vi "dfcg.vi"() -> ()   [LabVIEW 2020]
uses:
  <instrlib>/Lake Shore 372/Lake Shore 372.lvlib
panel:
  out "Quadrature Reading":dbl min=0.0 max=0.01 step=1e-05 format="%^.5e"
  out "Power Reading":dbl min=0.0 max=0.01 step=1e-05 format="%^.5e"
  out "Kelvin Reading":dbl min=0.0 max=1000.0 step=1e-05 format="%^.5e"
  out "Resistance Reading":dbl min=0.0 max=63200000.0 step=1e-05 format="%^.5e"
  in  "Channel (1:1)":u16(ring)=1 items=["1"=1, "2"=2, "3"=3, "4"=4, "5"=5, "6"=6, "7"=7, "8"=8, "9"=9, "10"=10, "11"=11, "12"=12, "13"=13, "14"=14, "15"=15, "16"=16, "A (Control Input)"=17]
  out "error out":errorcluster
  in  "VISA resource name":refnum<visa-resource-name>
  out "VISA resource name out":refnum<visa-resource-name>
  in  "error in (no error)":errorcluster
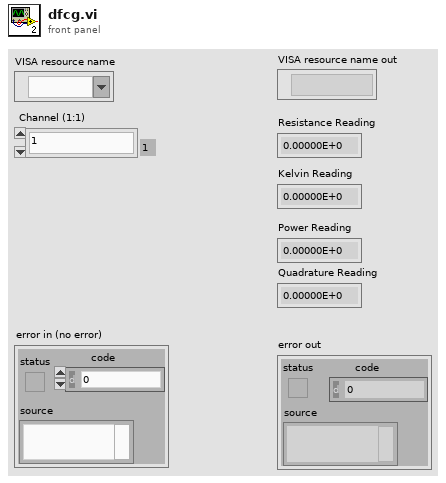
[diagram p1: front panel]
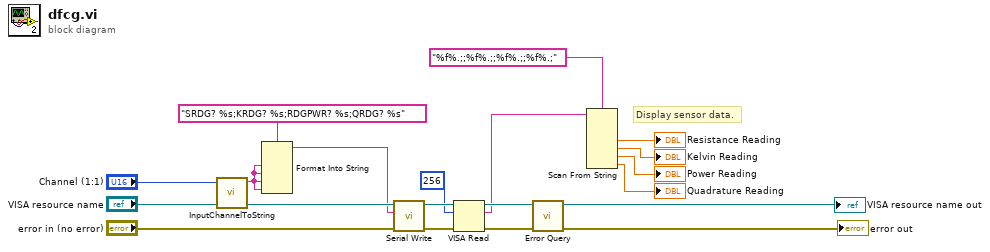
[diagram p0: block diagram]
diagram:
  # "Display sensor data."
  n1 = call <instrlib>:"InputChannelToString.vi"("Channel (1)"="Channel (1:1)") -> ("Channel Str"=w7:string)  [unwired: 10 in]
  n2 = Format Into String(format string="SRDG? %s;KRDG? %s;RDGPWR? %s;QRDG? %s", w7, w7, w7, w7) -> (resulting string=w5:string)  [unwired: 2 in, 1 out]
  n3 = call <instrlib>:"Serial Write.vi"("error in (no error)"="error in (no error)", "Write Buffer (\"\")"=w5, "VISA resource name"="VISA resource name") -> ("error out"=w6:errorcluster, "VISA resource name out"=w4:refnum<visa-resource-name>)  [unwired: 6 in, 1 out]
  n4 = VISA Read(VISA resource name=w4, byte count=u32 256, error in (no error)=w6) -> (VISA resource name out=w14:refnum<visa-resource-name>, read buffer=w3:string, error out=w2:errorcluster)  [unwired: 1 out]
  n5 = call <instrlib>:"Error Query.vi"("error in (no error)"=w2, "VISA resource name"=w14) -> ("error out"=→"error out":errorcluster, "VISA resource name out"=→"VISA resource name out":refnum<visa-resource-name>)  [unwired: 7 in, 1 out]
  n6 = Scan From String(format string="%f%.;;%f%.;;%f%.;;%f%.;", input string=w3) -> (output 1=→"Resistance Reading":dbl, output 2=→"Kelvin Reading":dbl, output 3=→"Power Reading":dbl, output 4=→"Quadrature Reading":dbl)  [unwired: 6 in, 3 out]
